vi "Draw 3D plane pos (1).vi"(7 "3D picture ref":refnum<vi>, 8 "Modify object":refnum<vi>, 9 "Draw object":refnum<vi>, 11 "Pos cluster ref":refnum<vi>) -> ()   [LabVIEW 2017]
uses:
  <userlib>/_MGI/Numeric/Coercion/MGI Degrees to Radians/MGI Degrees to Radians DBL.vi
  <vilib>/picture/3D Picture Control/NI_3D Picture Control.lvlib
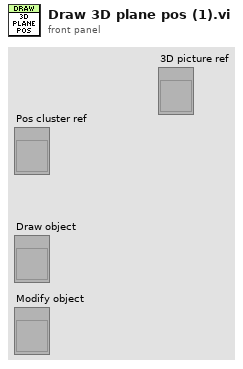
[diagram p1: front panel]
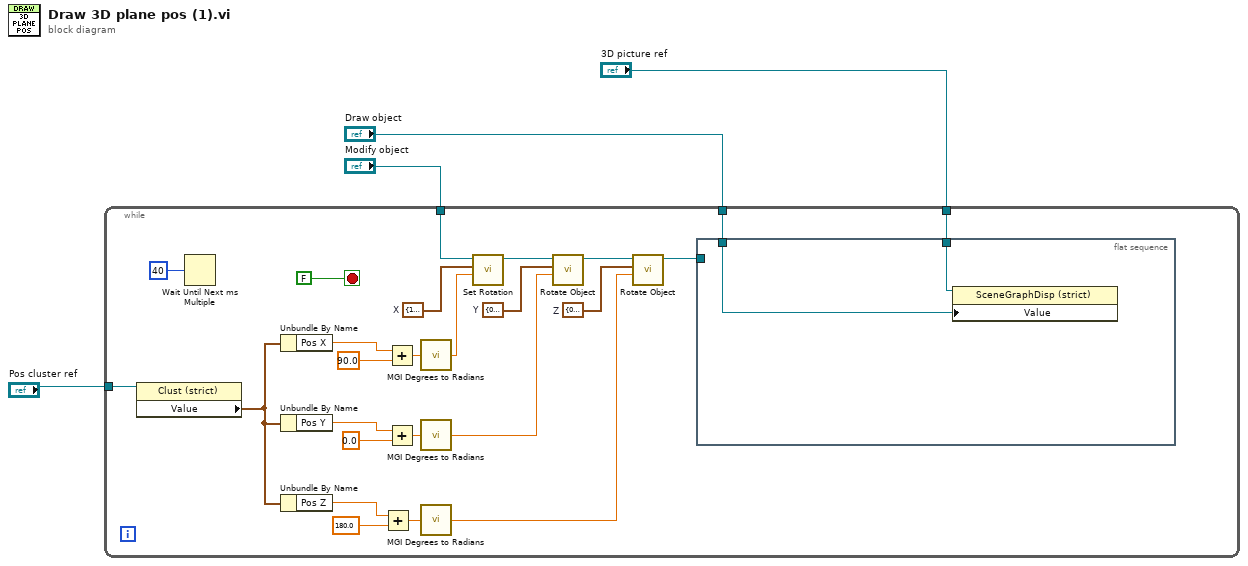
[diagram p0: block diagram]
diagram:
  n1 = while {
    tunnel: "Modify object" -> [w26]
    tunnel: "Draw object" -> [w25]
    tunnel: "Pos cluster ref" -> [w8]
    tunnel: "3D picture ref" -> [w5]
    stop <- FALSE stop-if-true
    w22 = cluster{"X":sgl, "Y":sgl, "Z":sgl} {"X"=0.0, "Y"=0.0, "Z"=1.0}  # Z
    w23 = cluster{"X":sgl, "Y":sgl, "Z":sgl} {"X"=0.0, "Y"=1.0, "Z"=0.0}  # Y
    w29 = cluster{"X":sgl, "Y":sgl, "Z":sgl} {"X"=1.0, "Y"=0.0, "Z"=0.0}  # X
    n2 = property class="Clust (strict)"(reference=w8) -> ("Value"=w7:cluster{"Pos X":dbl, "Pos Y":dbl, "Pos Z":dbl})  [unwired: 1 in, 2 out]
    n3 = Wait Until Next ms Multiple(millisecond multiple=u32 40 ("milliseconds to wait")) -> ()  [unwired: 1 out]
    n4 = Unbundle By Name(w7) -> ("Pos X"=w11:dbl)
    n5 = Unbundle By Name(w7) -> ("Pos Y"=w10:dbl)
    n6 = Unbundle By Name(w7) -> ("Pos Z"=w9:dbl)
    n7 = Add(x=w9, y=180.0) -> (x+y=w18:dbl)
    n8 = Add(x=w11, y=90.0) -> (x+y=w14:dbl)
    n9 = Add(x=w10, y=0.0) -> (x+y=w17:dbl)
    n10 = call-poly <userlib>:"MGI Degrees to Radians.vi"("Degrees"=w14) -> ("Radians"=w27:dbl)
    n11 = call-poly <userlib>:"MGI Degrees to Radians.vi"("Degrees"=w17) -> ("Radians"=w24:dbl)
    n12 = call-poly <userlib>:"MGI Degrees to Radians.vi"("Degrees"=w18) -> ("Radians"=w21:dbl)
    n13 = call <vilib>:"Set Rotation.vi"("Angle"=w27, "Axis"=w29, "Scene Object"=w26) -> ("Rotated Scene Object"=w20:refnum<vi>)  [unwired: 7 in, 1 out]
    n14 = call <vilib>:"Rotate Object.vi"("Angle"=w24, "Axis"=w23, "Scene.Object In"=w20) -> ("Scene.Object Out"=w19:refnum<vi>)  [unwired: 7 in, 1 out]
    n15 = call <vilib>:"Rotate Object.vi"("Angle"=w21, "Axis"=w22, "Scene.Object In"=w19) -> ("Scene.Object Out"=w12:refnum<vi>)  [unwired: 7 in, 1 out]
    n16 = flat-sequence {
      tunnel: w25 -> [w30]
      tunnel: w12 -> [_]
      tunnel: w5 -> [w31]
      frame #0 {
        n17 = property class="SceneGraphDisp (strict)"(reference=w31, "Value"=w30) -> ()  [unwired: 1 in, 2 out]
      }
    }
  }
